vi "Configure Sweep.vi"(0 "VISA resource name":refnum<visa-resource-name>, 1 "Enable Sweep (F: Disable)":bool, 2 "Sweep Start (0)":dbl, 3 "Sweep Number of Steps (1)":i32=1, 5 "Channel (0: Channel 1)":i32(ring) items=["Channel 1", "Channel 2"], 9 "Sweep Setting Mode (1: Voltage)":i32(ring)=1 items=["Current", "Voltage"], 11 "error in (no error)":errorcluster, 12 "Sweep Direction (0: Up)":i32(ring) items=["Up", "Down"], 13 "Sweep Stop (0)":dbl, 14 "Sweep Output Mode (0: Linear Single)":i32(ring) items=["Linear Single", "Linear Double", "Log Single", "Log Double"]) -> (4 "VISA resource name out":refnum<visa-resource-name>, 15 "error out":errorcluster)   [LabVIEW 2020, in "Agilent B2900 Series.lvlib"]
doc: "Configures sweep for measurement and source.\nOutput Mode control to select current or voltage mode to apply settings."
uses:
  Agilent B2900 Series.lvlib
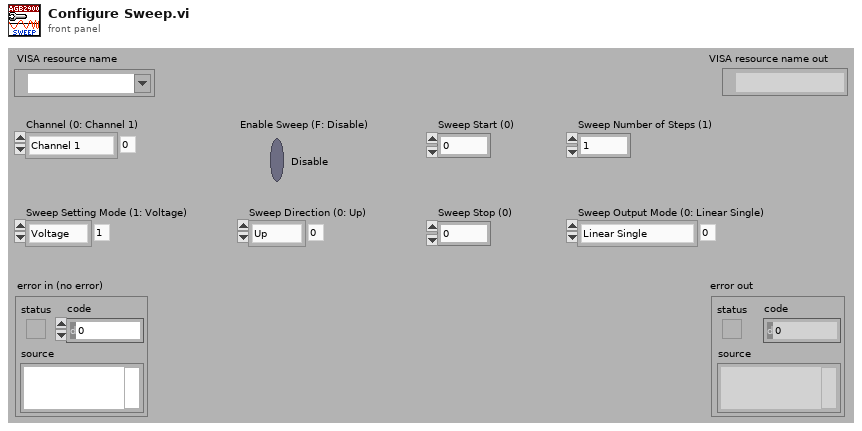
[diagram p1: front panel]
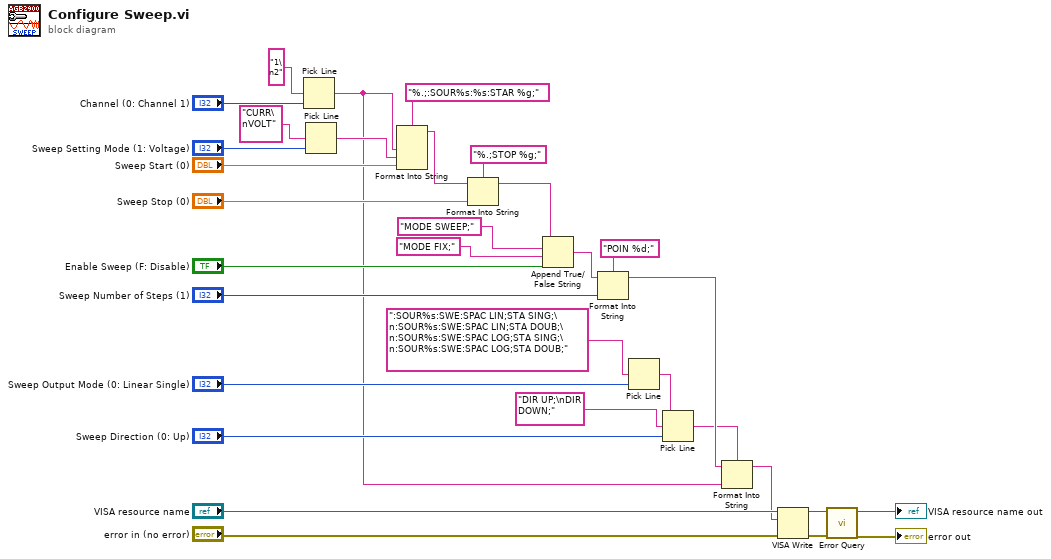
[diagram p0: block diagram]
diagram:
  n1 = Pick Line(multi-line string="1\n2" ("string (\"\")"), line index="Channel (0: Channel 1)") -> (output string=w2:string)  [unwired: 1 in]
  n2 = Pick Line(multi-line string="CURR\nVOLT" ("string (\"\")"), line index="Sweep Setting Mode (1: Voltage)") -> (output string=w6:string)  [unwired: 1 in]
  n3 = Format Into String(format string="%.;:SOUR%s:%s:STAR %g;", w2, w6, "Sweep Start (0)") -> (resulting string=w31:string)  [unwired: 2 in, 1 out]
  n4 = Format Into String(format string="%.;STOP %g;", initial string=w31, "Sweep Stop (0)") -> (resulting string=w28:string)  [unwired: 1 in, 1 out]
  n5 = Append True/False String(1:"Enable Sweep (F: Disable)", 2:"MODE FIX;", 3:"MODE SWEEP;", 4:w28) -> (0:w24:string)
  n6 = Format Into String(format string="POIN %d;", initial string=w24, "Sweep Number of Steps (1)") -> (resulting string=w4:string)  [unwired: 1 in, 1 out]
  n7 = Pick Line(multi-line string=":SOUR%s:SWE:SPAC LIN;STA SING;\n:SOUR%s:SWE:SPAC LIN;STA DOUB;\n:SOUR%s:SWE:SPAC LOG;STA SING;\n:SOUR%s:SWE:SPAC LOG;STA DOUB;", line index="Sweep Output Mode (0: Linear Single)") -> (output string=w5:string)  [unwired: 1 in]
  n8 = Pick Line(string ("")=w5, multi-line string="DIR UP;\nDIR DOWN;", line index="Sweep Direction (0: Up)") -> (output string=w3:string)
  n9 = Format Into String(format string=w3, initial string=w4, w2) -> (resulting string=w1:string)  [unwired: 1 in, 1 out]
  n10 = VISA Write(VISA resource name="VISA resource name", write buffer=w1, error in (no error)="error in (no error)") -> (VISA resource name out=w15:refnum<visa-resource-name>, error out=w14:errorcluster)  [unwired: 1 out]
  n11 = call "Error Query.vi"("error in (no error)"=w14, "VISA resource name"=w15) -> ("error out"=→"error out":errorcluster, "VISA resource name out"=→"VISA resource name out":refnum<visa-resource-name>)  [unwired: 6 in, 2 out]
